vi "Set average acquisition mode.vi"(8 "error in (no error)":errorcluster, 9 "NumberOfAverages":i32=500, 11 "IVI Refnum in":refnum<k15>) -> (0 "error out":errorcluster, 2 "log string out":string, 3 "IVI Refnum out":refnum<k15>)   [LabVIEW 2021]
uses:
  <instrlib>/Keysight InfiniiVision/Keysight InfiniiVision.lvlib
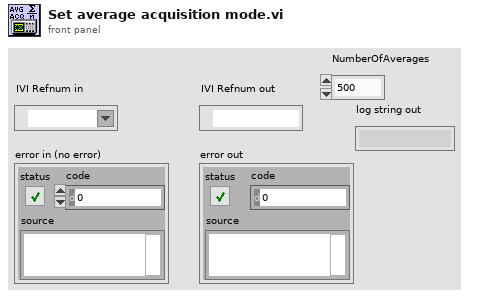
[diagram p1: front panel]
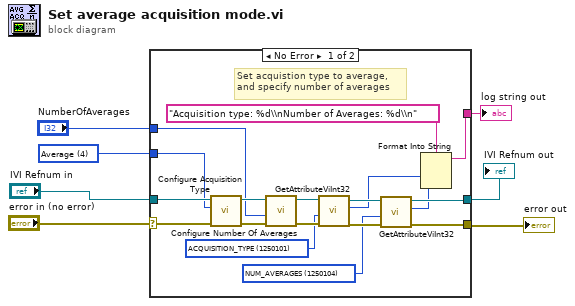
[diagram p0: block diagram]
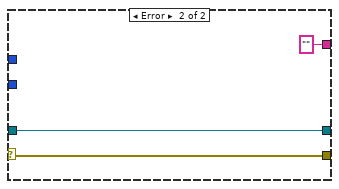
[diagram p2: hidden frame]
diagram:
  w3 = 4 items=["Normal", "Peak Detect", "High Resolution", "Envelope", "Average"] ("acquisition type (Normal)")
  n1 = case shown="No Error" "error in (no error)" {
    selector: "error in (no error)" -> [w22 w27]
    tunnel: [w13 w27] -> w7
    tunnel: [w14 w28] -> w6
    tunnel: "IVI Refnum in" -> [w25 w28]
    tunnel: w3 -> [w21 _]
    tunnel: "NumberOfAverages" -> [w20 _]
    tunnel: [w8 ""] -> w1
    frame No Error {
      w12 = u32 1250104 items=["AC_LINE_TRIGGER_SLOPE"=1250701, "ACQUISITION_SEGMENTEDMEMORY_INDEX"=1150139, "ACQUISITION_SEGMENTEDMEMORY_SEGMENT_COUNT"=1150138, "ACQUISITION_TYPE"=1250101, "CHANNEL_COUNT"=1050203, "CHANNEL_PROTECTION"=1150202, "CHANNEL_UNITS"=1150033, "DIGITALCHANNEL_COUNT"=1150038, "DIGITALCHANNEL_POSITION"=1150041, "DIGITALCHANNEL_SIZE"=1150042, "DVM_MODE"=1150443, "EXTERNAL_UNITS"=1150014, "GLITCH_CONDITION"=1250403, "GLITCH_POLARITY"=1250402, "HORZ_MIN_NUM_PTS"=1250009, "HORZ_RECORD_LENGTH"=1250008, "INTERPOLATION"=1250019, "NUM_AVERAGES"=1250104, "NUM_ENVELOPES"=1250105, "REFERENCE_SIGNAL"=1150433, "RUNT_POLARITY"=1250303, "SAMPLE_MODE"=1250106, "STATISTICS_FORMAT"=1150355, "STATUS_SERIAL_POLL"=1150019, "SYSTEM_IO_TIMEOUT"=1150607, "SYSTEM_PRECISION_RECORD_LENGTH"=1150589, "SYSTEM_TIMEOUT_MILLISECONDS"=1150023, "TIMEBASE_MODE"=1150107, "TIMEBASE_TIME_REFERENCE"=1150110, "TRIGGER_ACLINE_SLOPE"=1150556, "TRIGGER_COUPLING"=1250014, "TRIGGER_DELAY_ARMING_SLOPE"=1150263, "TRIGGER_DELAY_EDGE_COUNT"=1150267, "TRIGGER_DELAY_SLOPE"=1150266, "TRIGGER_EDGE_BURST_NTH_EDGE"=1150247, "TRIGGER_EDGE_BURST_SLOPE"=1150249, "TRIGGER_EDGE_REJECT_FILTER_TYPE"=1150135, "TRIGGER_MODIFIER"=1250102, "TRIGGER_PATTERN_CONDITION"=1150195, "TRIGGER_RUNT_CONDITION"=1150189, "TRIGGER_SETUP_AND_HOLD_SLOPE"=1150250, "TRIGGER_SLOPE"=1250018, "TRIGGER_TRANSITION_CONDITION"=1150255, "TRIGGER_TRANSITION_SLOPE"=1150256, "TRIGGER_TYPE"=1250012, "TRIGGER_TYPE_AG"=1150557, "TRIGGER_WIDTH_CONDITION"=1150197, "TRIGGER_WIDTH_POLARITY"=1150200, "VERTICAL_COUPLING"=1250003, "WAVEFORM_BYTE_ORDER"=1150085, "WAVEFORM_DATA_FORMAT"=1150086, "WAVEFORM_POINT_COUNT"=1150141, "WAVEFORM_POINT_MODE"=1150087, "WAVEFORM_SUB_SOOURCE"=1150609, "WAVEFORM_X_REFERENCE"=1150145, "WAVEFORM_Y_REFERENCE"=1150146, "WIDTH_CONDITION"=1250504, "WIDTH_POLARITY"=1250503] ("AttributeID")
      w17 = u32 1250101 items=["AC_LINE_TRIGGER_SLOPE"=1250701, "ACQUISITION_SEGMENTEDMEMORY_INDEX"=1150139, "ACQUISITION_SEGMENTEDMEMORY_SEGMENT_COUNT"=1150138, "ACQUISITION_TYPE"=1250101, "CHANNEL_UNITS"=1150033, "DIGITALCHANNEL_POSITION"=1150041, "DIGITALCHANNEL_SIZE"=1150042, "DVM_MODE"=1150443, "EXTERNAL_UNITS"=1150014, "GLITCH_CONDITION"=1250403, "GLITCH_POLARITY"=1250402, "HORZ_MIN_NUM_PTS"=1250009, "INTERPOLATION"=1250019, "NUM_AVERAGES"=1250104, "NUM_ENVELOPES"=1250105, "REFERENCE_SIGNAL"=1150433, "RUNT_POLARITY"=1250303, "STATISTICS_FORMAT"=1150355, "SYSTEM_IO_TIMEOUT"=1150607, "SYSTEM_PRECISION_RECORD_LENGTH"=1150589, "SYSTEM_TIMEOUT_MILLISECONDS"=1150023, "TIMEBASE_MODE"=1150107, "TIMEBASE_TIME_REFERENCE"=1150110, "TRIGGER_ACLINE_SLOPE"=1150556, "TRIGGER_COUPLING"=1250014, "TRIGGER_DELAY_ARMING_SLOPE"=1150263, "TRIGGER_DELAY_EDGE_COUNT"=1150267, "TRIGGER_DELAY_SLOPE"=1150266, "TRIGGER_EDGE_BURST_NTH_EDGE"=1150247, "TRIGGER_EDGE_BURST_SLOPE"=1150249, "TRIGGER_EDGE_REJECT_FILTER_TYPE"=1150135, "TRIGGER_MODIFIER"=1250102, "TRIGGER_PATTERN_CONDITION"=1150195, "TRIGGER_RUNT_CONDITION"=1150189, "TRIGGER_SETUP_AND_HOLD_SLOPE"=1150250, "TRIGGER_SLOPE"=1250018, "TRIGGER_TRANSITION_CONDITION"=1150255, "TRIGGER_TRANSITION_SLOPE"=1150256, "TRIGGER_TYPE"=1250012, "TRIGGER_TYPE_AG"=1150557, "TRIGGER_WIDTH_CONDITION"=1150197, "TRIGGER_WIDTH_POLARITY"=1150200, "VERTICAL_COUPLING"=1250003, "WAVEFORM_BYTE_ORDER"=1150085, "WAVEFORM_DATA_FORMAT"=1150086, "WAVEFORM_POINT_COUNT"=1150141, "WAVEFORM_POINT_MODE"=1150087, "WAVEFORM_SUB_SOOURCE"=1150609, "WIDTH_CONDITION"=1250504, "WIDTH_POLARITY"=1250503] ("AttributeID")
      # "Set acquistion type to average, \nand specify number of averages"
      n2 = call <instrlib>:"Configure Acquisition Type.vi"("error in (no error)"=w22, "acquisition type (Normal)"=w21, "instrument handle"=w25) -> ("error out"=w24:errorcluster, "instrument handle out"=w23:refnum<k15>)  [unwired: 7 in]
      n3 = call <instrlib>:"Configure Number Of Averages.vi"("error in (no error)"=w24, "NumberOfAverages"=w20, "instrument handle"=w23) -> ("error out"=w19:errorcluster, "instrument handle out"=w18:refnum<k15>)  [unwired: 7 in]
      n4 = call <instrlib>:"GetAttributeViInt32.vi"("error in (no error)"=w19, "AttributeID"=w17, "instrument handle"=w18) -> ("error out"=w15:errorcluster, "AttributeValue"=w10:i32, "instrument handle out"=w16:refnum<k15>)  [unwired: 6 in]
      n5 = call <instrlib>:"GetAttributeViInt32.vi"("error in (no error)"=w15, "AttributeID"=w12, "instrument handle"=w16) -> ("error out"=w13:errorcluster, "AttributeValue"=w11:i32, "instrument handle out"=w14:refnum<k15>)  [unwired: 6 in]
      n6 = Format Into String(format string="Acquisition type: %d\\nNumber of Averages: %d\\n", w10, w11) -> (resulting string=w8:string)  [unwired: 2 in, 1 out]
    }
    frame Error {
    }
  }
  "error out" <- w7
  "IVI Refnum out" <- w6
  "log string out" <- w1
